vi "write to file.vi"(0 "String":string="*50-*/", 1 "Boolean":bool) -> ()   [LabVIEW 2018]
panel:
  in  "show patch":bool
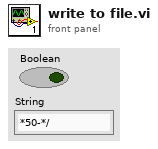
[diagram p1: front panel]
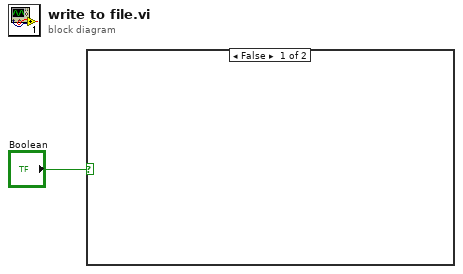
[diagram p0: block diagram]
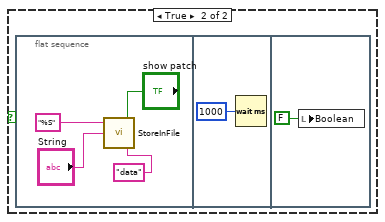
[diagram p2: hidden frame]
diagram:
  n1 = case shown="False" "Boolean" {
    frame False {
    }
    frame True {
      n2 = flat-sequence {
        frame #0 {
          n3 = call "StoreInFile.vi"("FileName"="data", "show patch"="show patch", "String"="String", "format"="%S") -> ()  [unwired: 1 in]
        }
        frame #1 {
          n4 = Wait (ms)(milliseconds to wait=u32 1000) -> ()  [unwired: 1 out]
        }
        frame #2 {
          n5 = local write "Boolean"(FALSE ("Boolean")) -> ()
        }
      }
    }
  }
